vi "FTW-Endpoint-Ask-Pipe.vi"(0 "FTW Endpoint":refnum<class "FTW-Endpoint.lvclass">, 5 "Request Header":string, 7 "Request Body":string, 9 "Timeout":i32=1000 format="%dmsec", 11 "error in":errorcluster) -> (4 "FTW Endpoint out":refnum<class "FTW-Endpoint.lvclass">, 6 "Response Header":string, 8 "Response Body":string, 10 "Timed out?":bool, 14 "Roundtrip Time":dbl format="%.6fsec", 15 "error out":errorcluster)   [LabVIEW 2013, in "FTW-Endpoint.lvclass"]
uses:
  FTW-Endpoint.lvclass
panel:
  # "Inputs"
  # "Outputs"
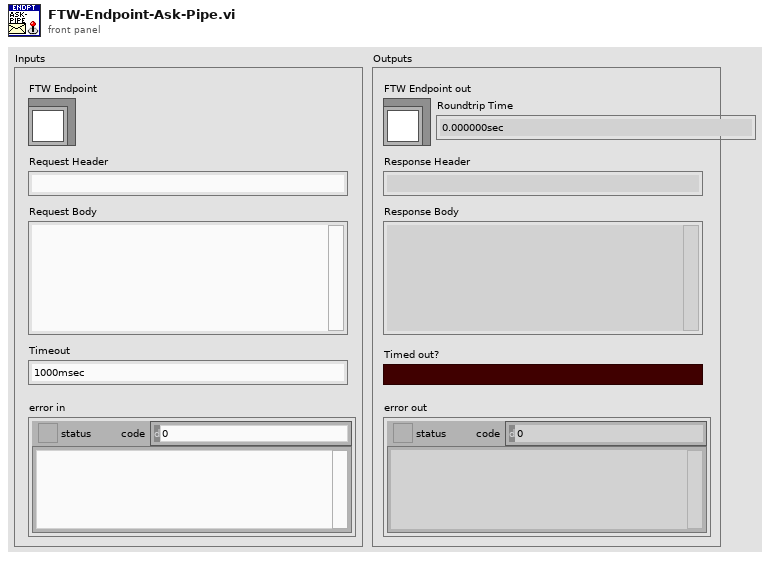
[diagram p1: front panel]
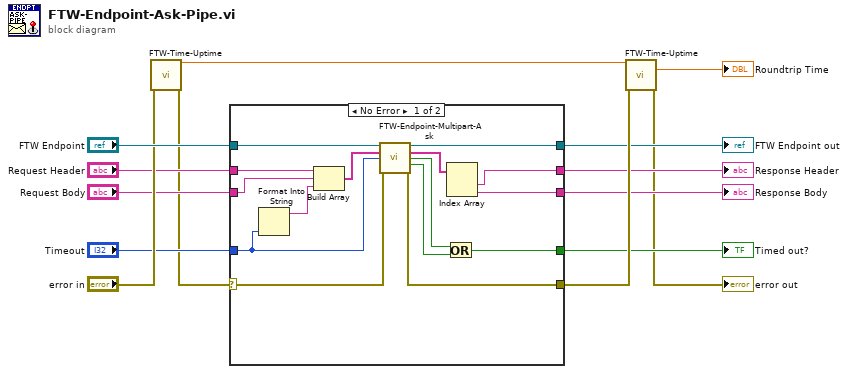
[diagram p0: block diagram]
diagram:
  n1 = call "FTW-Time-Uptime.vi"("error in"="error in") -> ("Current Uptime"=w2:dbl, "error out"=w4:errorcluster)  [unwired: 12 in, 1 out]
  n2 = case shown="No Error" w4 {
    selector: w4 -> [w25 w31]
    tunnel: [w24 w31] -> w14
    tunnel: [w26 w30] -> w12
    tunnel: "FTW Endpoint" -> [w27 w30]
    tunnel: [w20 _] -> w10
    tunnel: "Timeout" -> [w16 _]
    tunnel: "Request Header" -> [w29 _]
    tunnel: "Request Body" -> [w28 _]
    tunnel: [w18 _] -> w6
    tunnel: [w17 _] -> w5
    frame No Error {
      n3 = Format Into String(w16) -> (resulting string=w15:string)  [unwired: 3 in, 1 out]
      n4 = Build Array(w29, w28, w15) -> (w23:string[])
      n5 = call-dynamic "FTW-Endpoint-Multipart-Ask.vi"("FTW Endpoint"=w27, "Multipart Message"=w23, "Read Timeout"=w16, "error in"=w25) -> ("FTW Endpoint out"=w26:refnum<class "FTW-Endpoint.lvclass">, "Reply"=w19:string[], "Read Timed out?"=w22:bool, "Write Timed out?"=w21:bool, "error out"=w24:errorcluster)  [unwired: 7 in]
      n6 = Or(x=w22, y=w21) -> (x .or. y?=w20:bool)
      n7 = Index Array(array=w19) -> (element #1=w18:string, element #2=w17:string)  [unwired: 2 in]
    }
    frame Error {
    }
  }
  "FTW Endpoint out" <- w12
  "Timed out?" <- w10
  "Response Header" <- w6
  "Response Body" <- w5
  n8 = call "FTW-Time-Uptime.vi"("Previous Uptime"=w2, "error in"=w14) -> ("Elapsed Time"=→"Roundtrip Time":dbl, "error out"=→"error out":errorcluster)  [unwired: 11 in, 1 out]
